vi "Meas Result Generate TWM Digitizer Correction - Estimate Digitizer Uncertainty.vi"(9 "Estimate non-linearity (False)":bool, 10 "digitizer type":T1=enum."HP3458A", 11 "correction data in":T2) -> (3 "correction data out":T2)   [LabVIEW 2020]
doc: "Very crude estimation of nonlinearity errors of selected digitizer type."
uses:
  Meas Results TWM Digitizer Correction Data.ctl
  results/Meas Results Correction Structuring Mode.ctl
  Meas Results TWM Correction Digitizer Type.ctl
panel:
  out "output array":dbl[][][](array[numeric])
  in  "Array":dbl[][](array[numeric])
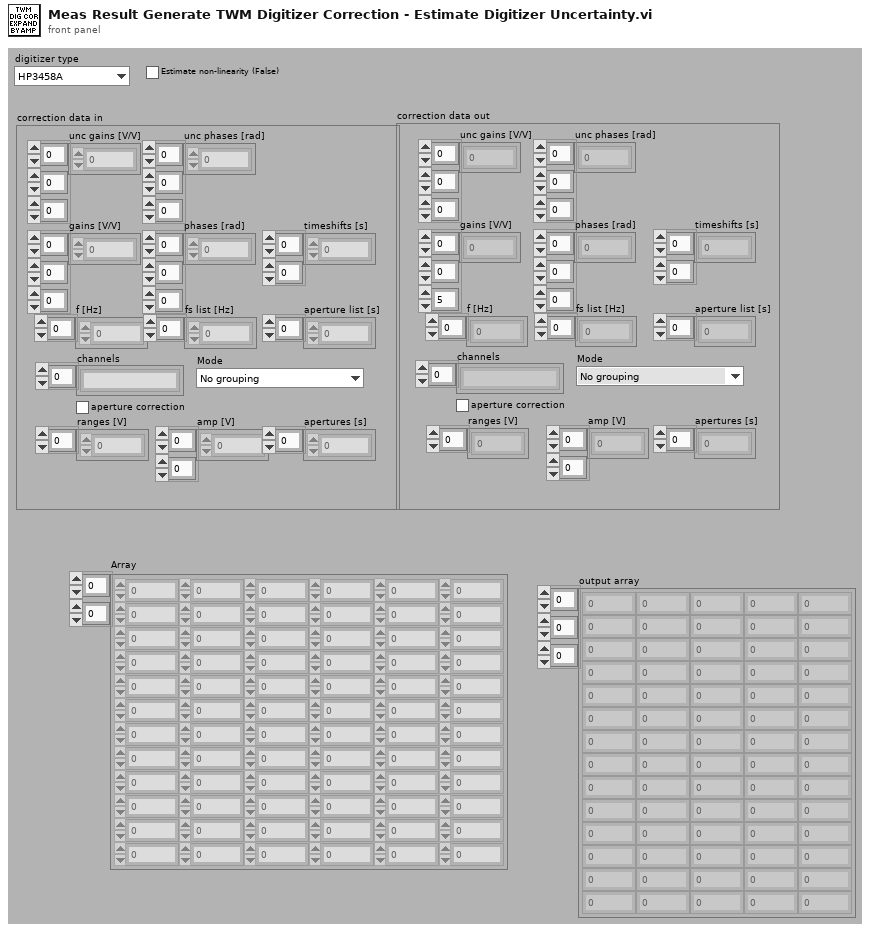
[diagram p1: front panel]
types:
  T1 = typedef "Meas Results TWM Correction Digitizer Type.ctl" = enum16{"Unknown", "HP3458A", "NI9238"}
  T2 = typedef "Meas Results TWM Digitizer Correction Data.ctl" = cluster{"gains [V/V]":dbl[][][], "phases [rad]":dbl[][][], "timeshifts [s]":dbl[][], "f [Hz]":dbl[], "fs list [Hz]":dbl[], "aperture list [s]":dbl[], "channels":string[], "Mode":T3, "aperture correction":bool, "ranges [V]":dbl[], "amp [V]":dbl[][], "apertures [s]":dbl[], "unc gains [V/V]":dbl[][][], "unc phases [rad]":dbl[][][]}
  T3 = typedef "Meas Results Correction Structuring Mode.ctl" = enum16{"No grouping", "Group by apertures (3458A)", "Group by fs (generic digitizer)"}
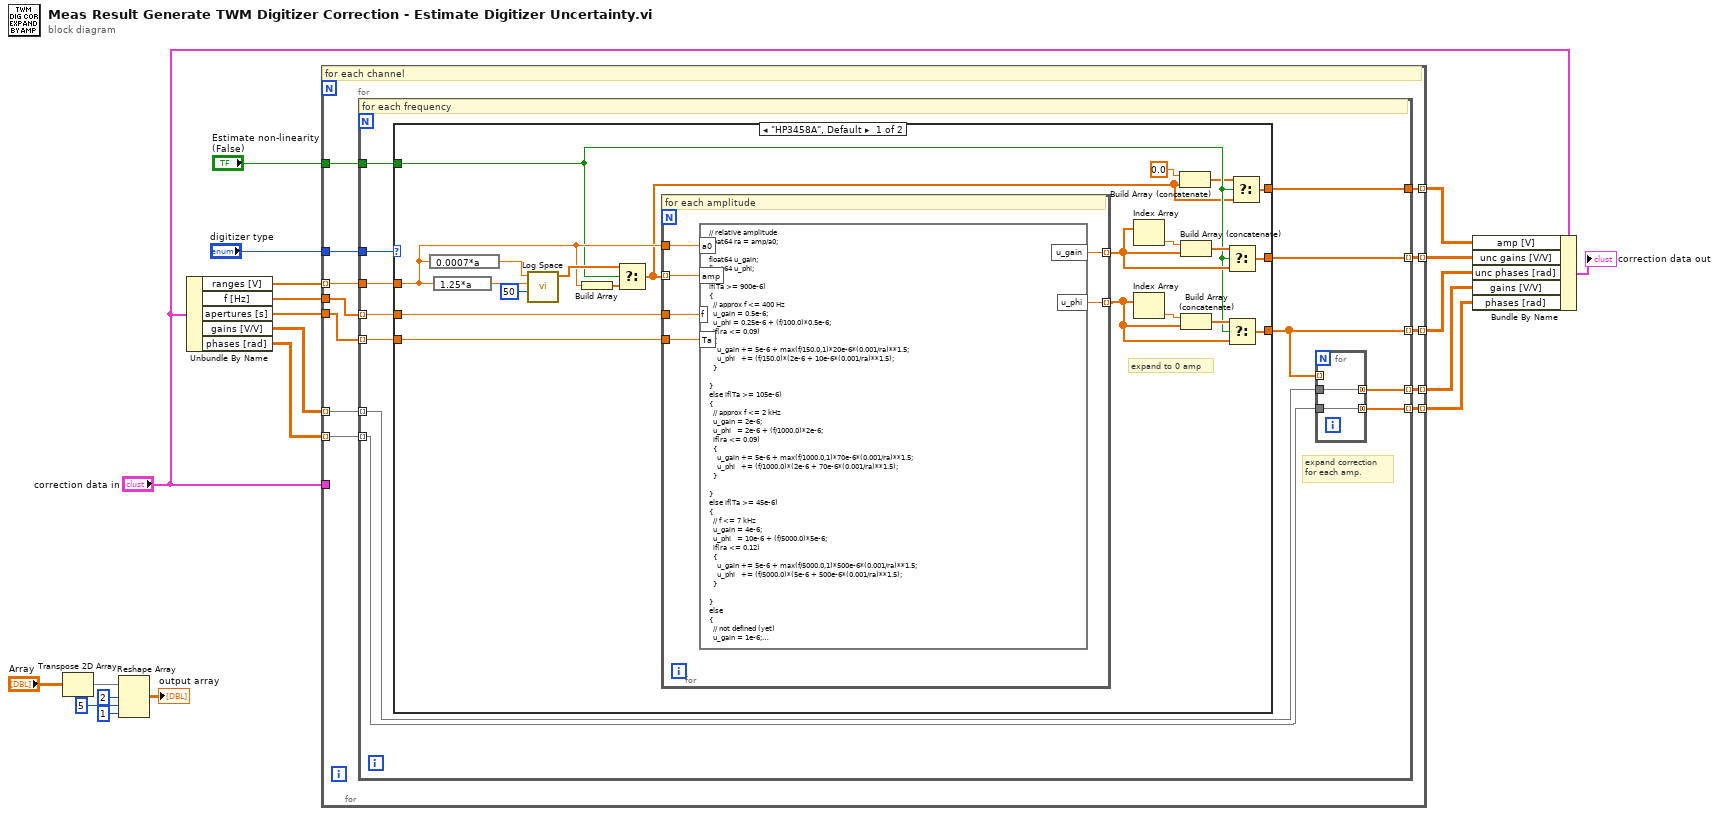
[diagram p0: block diagram]
diagram:
  n1 = Transpose 2D Array(2D array="Array") -> (transposed array=w11:dbl[][])
  n2 = Reshape Array(w11, 2 ("dimension size"), 5 ("dimension size"), 1 ("dimension size")) -> (→"output array":dbl[][][])
  n3 = Unbundle By Name("correction data in") -> ("ranges [V]"=w17:dbl[], "f [Hz]"=w20:dbl[], "apertures [s]"=w19:dbl[], "gains [V/V]"=w10:dbl[][][], "phases [rad]"=w9:dbl[][][])
  n4 = for {
    tunnel: "correction data in" -> [_]
    tunnel: w10 -> [w32] mode=indexing
    tunnel: w9 -> [w31] mode=indexing
    tunnel: w20 -> [w28]
    tunnel: w19 -> [w27]
    tunnel: "digitizer type" -> [w30]
    tunnel: w17 -> [w29] mode=indexing
    tunnel: [w26] -> w7 mode=indexing
    tunnel: [w25] -> w6 mode=indexing
    tunnel: "Estimate non-linearity (False)" -> [w24]
    tunnel: [w23] -> w3 mode=indexing
    tunnel: [w22] -> w2 mode=indexing
    tunnel: [w21] -> w1 mode=indexing
    # "for each channel"
    n5 = for {
      tunnel: w32 -> [w37] mode=indexing
      tunnel: w31 -> [w34] mode=indexing
      tunnel: w30 -> [w44]
      tunnel: w29 -> [w43]
      tunnel: w28 -> [w42] mode=indexing
      tunnel: w27 -> [w41] mode=indexing
      tunnel: [w40] -> w26 mode=indexing
      tunnel: [w36] -> w25 mode=indexing
      tunnel: w24 -> [w39]
      tunnel: [w38] -> w23
      tunnel: [w35] -> w22 mode=indexing
      tunnel: [w33] -> w21 mode=indexing
      # "expand correction\nfor each amp."
      # "for each frequency"
      n6 = case shown="\"HP3458A\", Default" w44 {
        tunnel: w43 -> [w54 _]
        tunnel: w42 -> [w64 _]
        tunnel: w41 -> [w63 _]
        tunnel: [w60 _] -> w40
        tunnel: [w52 _] -> w36
        tunnel: w39 -> [w51 _]
        tunnel: [w49 _] -> w38
        frame "HP3458A", Default {
          # "expand to 0 amp"
          n7 = expression code="0.0007*a"(w54) -> (w65:dbl)
          n8 = expression code="1.25*a"(w54) -> (w66:dbl)
          n9 = call "Log Space.vi"("Number of Samples"=u32 50, "Maximum"=w66, "Minimum"=w65) -> ("Array"=w55:dbl[])  [unwired: 7 in, 1 out]
          n10 = Build Array(w54) -> (w53:dbl[])
          n11 = Select(t=w55, s=w51, f=w53) -> (s? t:f=w48:dbl[])
          n12 = for {
            tunnel: w48 -> [w73] mode=indexing
            tunnel: w64 -> [w72]
            tunnel: w63 -> [w71]
            tunnel: w54 -> [w70]
            tunnel: [w69] -> w57 mode=indexing
            tunnel: [w68] -> w56 mode=indexing
            # "for each amplitude"
            n13 = formula code="// relative amplitude\nfloat64 ra = amp/a0;\n\nfloat64 u_gain;\nfloat64 u_phi;\n\nif(Ta >= 900e-6)\n{\n  // approx f <= 400 Hz\n  u_gain = 0.5e-6;\n  u_phi = 0.25e-6 + (f/100.0)*0.5e-6;\n  if(ra <= 0.09)\n  {\n    u_gain += 5e-6 + max(f/150.0,1)*20e-6*(0.001/ra)**1.5;\n    u_phi   += (f/150.0)*(2e-6 + 10e-6*(0.001/ra)**1.5);\n  }\n  \n}\nelse if(Ta >= 105e-6)\n{\n  // approx f <= 2 kHz\n  u_gain = 2e-6;\n  u_phi   = 2e-6 + (f/1000.0)*2e-6;\n  if(ra <= 0.09)\n  {\n    u_gain += 5e-6 + max(f/1000.0,1)*70e-6*(0.001/ra)**1.5;\n    u_phi   += (f/1000.0)*(2e-6 + 70e-6*(0.001/ra)**1.5);\n  }\n\n}\nelse if(Ta >= 45e-6)\n{\n  // f <= 7 kHz\n  u_gain = 4e-6;\n  u_phi   = 10e-6 + (f/5000.0)*5e-6;\n  if(ra <= 0.12)\n  {\n    u_gain += 5e-6 + max(f/5000.0,1)*500e-6*(0.001/ra)**1.5;\n    u_phi   += (f/5000.0)*(5e-6 + 500e-6*(0.001/ra)**1.5);\n  }\n\n}\nelse\n{\n  // not defined (yet)\n  u_gain = 1e-6;\n  u_phi = 0.5e-6;\n}\n\n// convert to k = 1\nu_gain *= 0.5;\nu_phi *= 0.5;"("amp"=w73, "f"=w72, "Ta"=w71, "a0"=w70) -> ("u_gain"=w69:dbl, "u_phi"=w68:dbl)
          }
          n14 = Index Array(array=w57) -> (element=w62:dbl)  [unwired: 1 in]
          n15 = Index Array(array=w56) -> (element=w61:dbl)  [unwired: 1 in]
          n16 = Build Array (concatenate)(0.0, w48) -> (w50:dbl[])
          n17 = Build Array (concatenate)(w62, w57) -> (w59:dbl[])
          n18 = Build Array (concatenate)(w61, w56) -> (w58:dbl[])
          n19 = Select(t=w59, s=w51, f=w57) -> (s? t:f=w60:dbl[])
          n20 = Select(t=w58, s=w51, f=w56) -> (s? t:f=w52:dbl[])
          n21 = Select(t=w50, s=w51, f=w48) -> (s? t:f=w49:dbl[])
        }
        frame "NI9238" {
        }
      }
      n22 = for {
        tunnel: w37 -> [w46]
        tunnel: w36 -> [_] mode=indexing
        tunnel: [w46] -> w35 mode=concatenating
        tunnel: [w45] -> w33 mode=concatenating
        tunnel: w34 -> [w45]
      }
    }
  }
  n23 = Bundle By Name(cluster="correction data in", "amp [V]"=w3, "unc gains [V/V]"=w7, "unc phases [rad]"=w6, "gains [V/V]"=w2, "phases [rad]"=w1) -> (→"correction data out":T2)
